vi "Read Single Digital Channel.vi"(8 "error in (no error)":errorcluster, 10 "Pin Number":T1(ring), 11 "VISA resource name":refnum<visa-resource-name>) -> (0 "error out":errorcluster, 2 "Pin State":bool, 3 "VISA resource name out":refnum<visa-resource-name>)   [LabVIEW 2020, in "BDAQ-6104.lvlib"]
uses:
  <instrlib>/BDAQ-6104/BDAQ-6104.lvlib
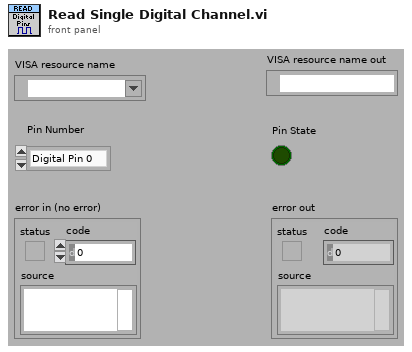
[diagram p1: front panel]
types:
  T1 = enum16{"Digital Pin 0", "Digital Pin 1", "Digital Pin 2", "Digital Pin 3"}
  T2 = cluster{"DIO0":bool, "DIO1":bool, "DIO2":bool, "DIO3":bool}
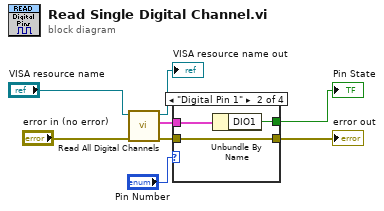
[diagram p0: block diagram]
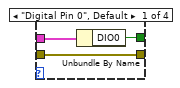
[diagram p2: hidden frame]
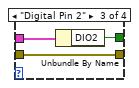
[diagram p3: hidden frame]
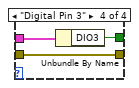
[diagram p4: hidden frame]
diagram:
  n1 = call <instrlib>:"Read All Digital Channels.vi"("error in (no error)"="error in (no error)", "VISA resource name"="VISA resource name") -> ("error out"=w3:errorcluster, "Digital Outputs"=w4:T2, "VISA resource name out"=→"VISA resource name out":refnum<visa-resource-name>)  [unwired: 6 in]
  n2 = case shown="\"Digital Pin 1\"" "Pin Number" {
    tunnel: w4 -> [w11 w14 w17 w20]
    tunnel: w3 -> [w9 w13 w15 w18]
    tunnel: [w9 w13 w15 w18] -> w1
    tunnel: [w10 w12 w16 w19] -> w2
    frame "Digital Pin 0", Default {
      n3 = Unbundle By Name(w11) -> ("DIO0"=w10:bool)
    }
    frame "Digital Pin 1" {
      n4 = Unbundle By Name(w14) -> ("DIO1"=w12:bool)
    }
    frame "Digital Pin 2" {
      n5 = Unbundle By Name(w17) -> ("DIO2"=w16:bool)
    }
    frame "Digital Pin 3" {
      n6 = Unbundle By Name(w20) -> ("DIO3"=w19:bool)
    }
  }
  "error out" <- w1
  "Pin State" <- w2
